vi "Init.vi"(9 "Event":refnum<class "Event jettl.lvclass">, 10 "Self Event Alias":string) -> (3 "Create Event Msg Strategy out":refnum<class "Create Event Msg Strategy.lvclass">)   [LabVIEW 2021, in "jettl Msg Create Event.lvlib" / "Create Event Msg Strategy.lvclass"]
uses:
  Create Event Msg Strategy.lvclass
  Create Event Msg Strategy.lvclass/Create Event Msg Strategy.ctl
  jettl/Event jettl/Event jettl.lvclass
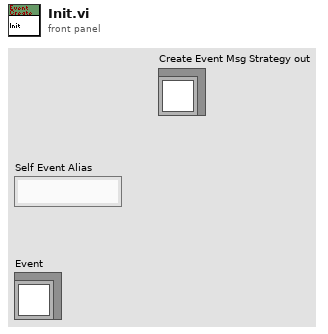
[diagram p1: front panel]
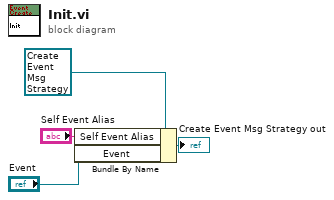
[diagram p0: block diagram]
diagram:
  n1 = Bundle By Name(cluster=refnum<class "Create Event Msg Strategy.lvclass"> refnum ("Event Create Msg out"), "Self Event Alias"="Self Event Alias", "Event"="Event") -> (→"Create Event Msg Strategy out":refnum<class "Create Event Msg Strategy.lvclass">)
